vi "generate random channels.vi"(9 "Supported Channel Classifications":T1[](array[typedef]), 10 "supported types":T2[](array[typedef]), 11 "Number of Random Channels to Create":i32) -> (3 "Random Channels":refnum<class "TBM channel.lvclass">[](array[class]))   [LabVIEW 2015, in "E2E Tag Exchange tests.lvlib"]
uses:
  E2E Tag Exchange tests.lvlib
  <vilib>/NI/Tag Bus/tag/Data Type.ctl
  <vilib>/NI/Tag Bus Module Framework/channel/channel classification.ctl
  <vilib>/NI/Tag Bus Module Framework/channel/TBM channel.lvclass
  <vilib>/NI/Tag Bus/tag/tag descriptor.lvclass
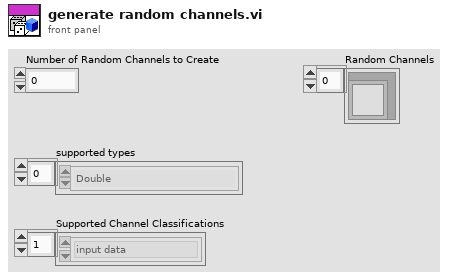
[diagram p1: front panel]
types:
  T1 = typedef "TBM channel.lvclass/channel classification.ctl" = enum16{"input data", "output data", "processing parameter", "processing result"}
  T2 = typedef "tag bus.lvlib/tag descriptor.lvclass/Data Type.ctl" = enum16{"Double", "Single", "I64", "I32", "I16", "I8", "U64", "U32", "U16", "U8", "Boolean", "String", "Array of Double", "Array of Single", "Array of I64", "Array of I32", "Array of I16", "Array of I8", "Array of U64", "Array of U32", "Array of U16", "Array of U8", "Array of Boolean", "Array of String"}
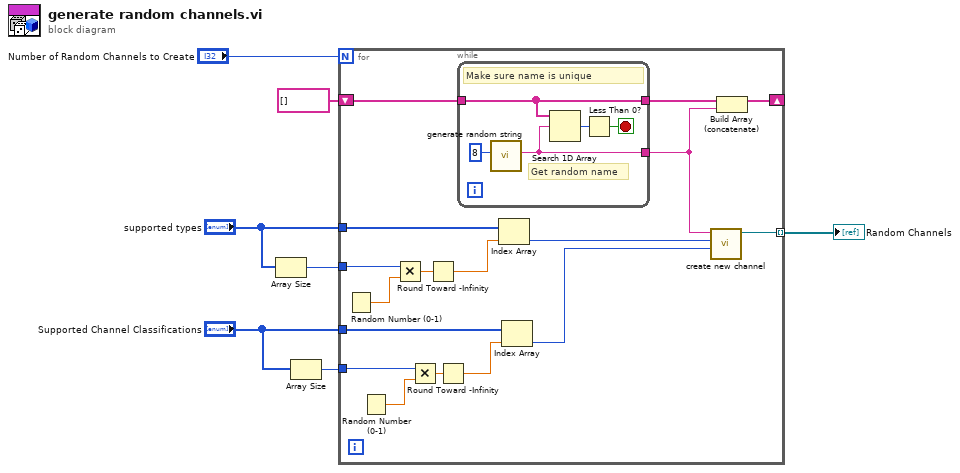
[diagram p0: block diagram]
diagram:
  n1 = Array Size(array="supported types") -> (size(s)=w6:i32)
  n2 = Array Size(array="Supported Channel Classifications") -> (size(s)=w3:i32)
  n3 = for {
    N: "Number of Random Channels to Create" -> [_]
    tunnel: "supported types" -> [w22]
    tunnel: w6 -> [w24]
    tunnel: "Supported Channel Classifications" -> [w19]
    tunnel: w3 -> [w18]
    shift-right: [w17] -> _
    shift-left: string[] [] -> [w16]
    tunnel: [w13] -> w2 mode=indexing
    n4 = Random Number (0-1)() -> (number: 0 to 1=w23:dbl)
    n5 = Random Number (0-1)() -> (number: 0 to 1=w20:dbl)
    n6 = Multiply(x=w24, y=w23) -> (x*y=w12:dbl)
    n7 = Multiply(x=w18, y=w20) -> (x*y=w11:dbl)
    n8 = Round Toward -Infinity(1:w12) -> (0:w9:dbl)
    n9 = Round Toward -Infinity(1:w11) -> (0:w8:dbl)
    n10 = while {
      tunnel: w16 -> [w29]
      tunnel: [w29] -> w15
      tunnel: [w26] -> w14
      stop <- w27 stop-if-true
      # "Get random name"
      # "Make sure name is unique"
      n11 = call "generate random string.vi"("Number of Characters"=8) -> ("string"=w26:string)  [unwired: 10 in]
      n12 = Search 1D Array(1D array=w29, element=w26) -> (index of element=w28:i32)  [unwired: 1 in]
      n13 = Less Than 0?(x=w28) -> (x < 0?=w27:bool)
    }
    n14 = Index Array(array=w22, index=w9) -> (element=w21:T2)
    n15 = Index Array(array=w19, index=w8) -> (element=w10:T1)
    n16 = call <vilib>:"create new channel.vi"("channel classification"=w10, "data type"=w21, "channel name"=w14) -> ("channel"=w13:refnum<class "TBM channel.lvclass">)  [unwired: 8 in]
    n17 = Build Array (concatenate)(w15, w14) -> (w17:string[])
  }
  "Random Channels" <- w2
